vi "BFS Index To Tag.vi"(9 "BFS Index In":i32[](array[numeric]), 11 "Root Tag In":string) -> (2 "Tag Out":string)   [LabVIEW 2022 SP3]
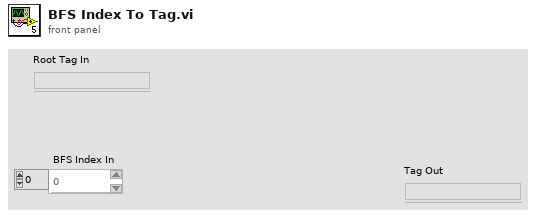
[diagram p1: front panel]
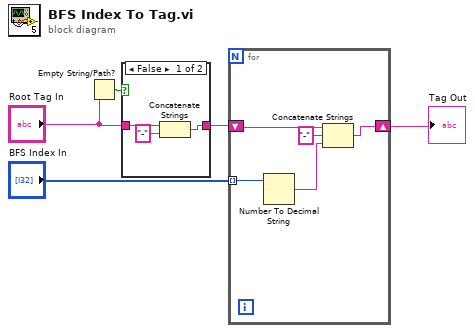
[diagram p0: block diagram]
diagram:
  n1 = Empty String/Path?(string/path="Root Tag In") -> (empty?=w5:bool)
  n2 = case shown="False" w5 {
    tunnel: "Root Tag In" -> [w8 w9]
    tunnel: [w6 w9] -> w3
    frame False {
      n3 = Concatenate Strings(w8, "-" ("string")) -> (w6:string)
    }
    frame True {
    }
  }
  n4 = for {
    shift-right: [w11] -> w1
    shift-left: w3 -> [w12]
    tunnel: "BFS Index In" -> [w14] mode=indexing
    n5 = Number To Decimal String(number=w14) -> (decimal integer string=w10:string)  [unwired: 1 in]
    n6 = Concatenate Strings(w12, "-" ("string"), w10) -> (w11:string)
  }
  "Tag Out" <- w1
